vi "GetSubVIs.vi"(6 "error in":errorcluster, 9 "Diagram in":refnum<class "Diagram.lvclass">) -> (0 "error out":errorcluster, 3 "Diagram out":refnum<class "Diagram.lvclass">, 4 "subVIs":i32[](array[numeric]))   [LabVIEW 2014, in "Diagram.lvclass"]
uses:
  Diagram.lvclass
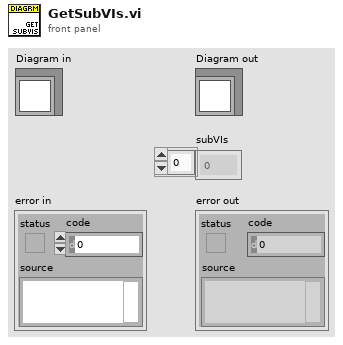
[diagram p1: front panel]
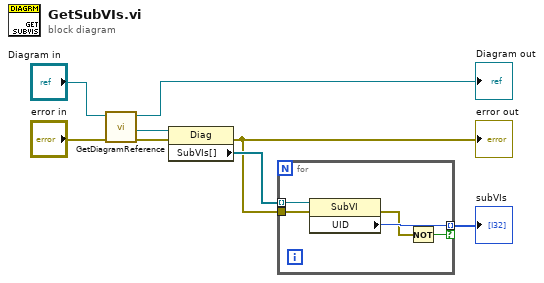
[diagram p0: block diagram]
diagram:
  n1 = call "GetDiagramReference.vi"("error in"="error in", "Diagram in"="Diagram in") -> ("error out"=w5:errorcluster, "reference out"=w4:refnum<vi>, "Diagram out"=→"Diagram out":refnum<class "Diagram.lvclass">)  [unwired: 5 in]
  n2 = property class="Diag"(reference=w4, error in=w5) -> (error out=w1:errorcluster, "SubVIs[]"=w3:refnum<vi>[])  [unwired: 1 out]
  "error out" <- w1
  n3 = for {
    tunnel: w3 -> [w10] mode=indexing
    tunnel: w1 -> [w9]
    tunnel: [w13] -> w2 mode=indexing if=w11
    n4 = property class="SubVI"(reference=w10, error in=w9) -> (error out=w12:errorcluster, "UID"=w13:i32)  [unwired: 1 out]
    n5 = Not(x=w12) -> (.not. x?=w11:bool)
  }
  "subVIs" <- w2
